vi "get WFS scan derived parameters.vi"(8 "error in (no error)":errorcluster, 11 "ImagingModeSPIM in":refnum<class "ImagingModeSPIM.lvclass">) -> (0 "error out":errorcluster, 3 "ImagingModeSPIM out":refnum<class "ImagingModeSPIM.lvclass">)   [LabVIEW 2012, in "ImagingModeSPIM.lvclass"]
uses:
  ImagingModeSPIM.lvclass
  Controls/waveform_enum.ctl
  ImagingModeSPIM.lvclass/ImagingModeSPIM.ctl
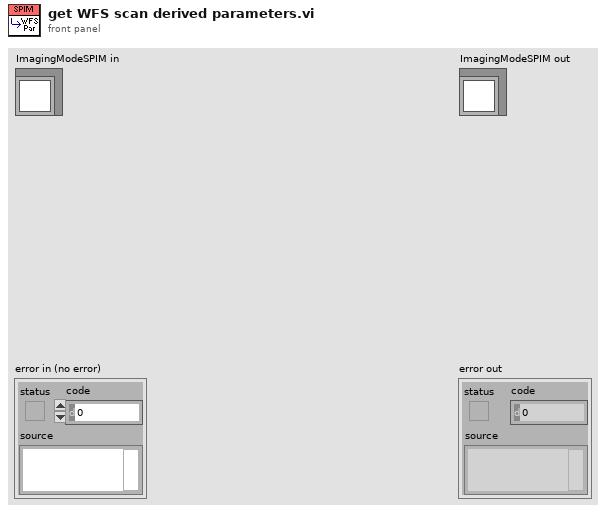
[diagram p1: front panel]
types:
  T1 = typedef "ImagingModeSPIM.lvclass/waveform_enum.ctl" = enum16{"triangular", "step", "sawtooth", "sinusodial", "skewed sawtooth"}
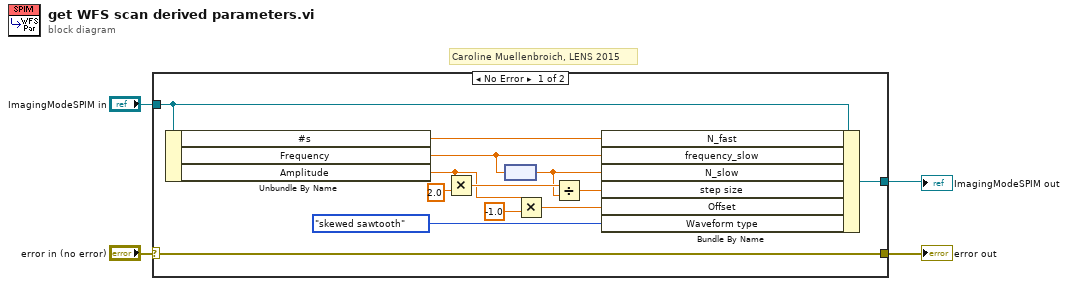
[diagram p0: block diagram]
diagram:
  # "Caroline Muellenbroich, LENS 2015"
  n1 = case shown="No Error" "error in (no error)" {
    selector: "error in (no error)" -> [w6 w19]
    tunnel: [w6 w19] -> w3
    tunnel: "ImagingModeSPIM in" -> [w17 w18]
    tunnel: [w5 w18] -> w1
    frame No Error {
      n2 = Unbundle By Name(w17) -> ("#s"=w14:dbl, "Frequency"=w12:dbl[unit], "Amplitude"=w8:dbl[unit])
      n3 = Multiply(x=w8, y=2.0) -> (x*y=w16:dbl[unit])
      n4 = node(w12) -> (w7:dbl)
      n5 = Multiply(x=w8, y=-1.0) -> (x*y=w10:dbl[unit])
      n6 = Divide(x=w16, y=w7) -> (x/y=w13:dbl[unit])
      n7 = Bundle By Name(cluster=w17, "N_fast"=w14, "frequency_slow"=w12, "N_slow"=w7, "step size"=w13, "Offset"=w10, "Waveform type"=waveform_enum."skewed sawtooth" ("y")) -> (w5:refnum<class "ImagingModeSPIM.lvclass">)
    }
    frame Error {
    }
  }
  "error out" <- w3
  "ImagingModeSPIM out" <- w1
